vi "Execute.vi"(8 "error in":errorcluster, 11 "Change O3 Generator State in":refnum<class "Change O3 Generator State.lvclass">) -> (0 "error out":errorcluster, 1 "Next Step?":bool, 2 "MSG":string, 3 "Change O3 Generator State out":refnum<class "Change O3 Generator State.lvclass">)   [LabVIEW 2015, in "Change O3 Generator State.lvclass"]
uses:
  Change O3 Generator State.lvclass
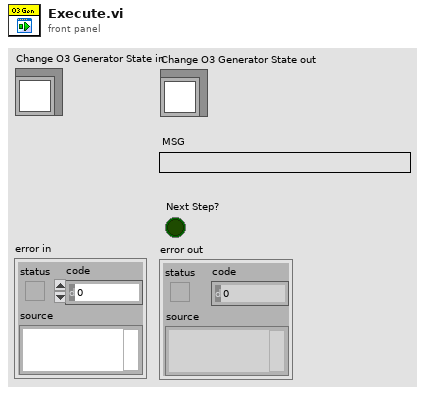
[diagram p1: front panel]
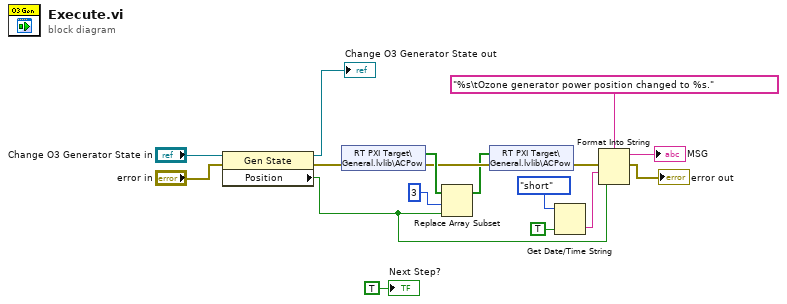
[diagram p0: block diagram]
diagram:
  n1 = property class="Gen State"(reference="Change O3 Generator State in", error in="error in") -> (reference out=→"Change O3 Generator State out":refnum<class "Change O3 Generator State.lvclass">, error out=w9:errorcluster, "Position"=w6:bool)
  n2 = shared-variable "RT PXI Target\\General.lvlib\\ACPow"(error in=w9) -> (w11:bool[], error out=w8:errorcluster)
  n3 = Replace Array Subset(array=w11, new element=w6, index=3) -> (w7:bool[])
  n4 = shared-variable "RT PXI Target\\General.lvlib\\ACPow"(w7, error in=w8) -> (error out=w12:errorcluster)
  n5 = Get Date/Time String(date format (0)=enum16{"short", "long", "abbreviated"}."short", want seconds? (F)=TRUE) -> (time string=w14:string)  [unwired: 1 in, 1 out]
  n6 = Format Into String(format string="%s\tOzone generator power position changed to %s.", error in=w12, w14, w6) -> (resulting string=→"MSG":string, error out=→"error out":errorcluster)  [unwired: 1 in]
  "Next Step?" <- TRUE ("Next Step?")
